vi "CODMn启动命令 (子VI).vi"(9 "强制切换":bool, 10 "CODMn量程切换":enum32{"H", "L", "AUTO"}(ring)=enum."AUTO", 11 "启动测量模式":T1) -> ()   [LabVIEW 2016, in "斯坦道CODMn.lvlib"]
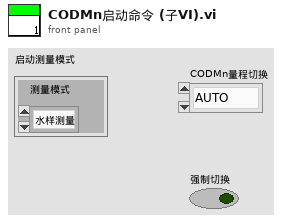
[diagram p1: front panel]
types:
  T1 = cluster{"测量模式":enum16{"水样测量", "标样核查", "零点核查", "跨度核查", "空白测试", "加标回收", "平行样", "校零", "校标"}}
  T2 = cluster{"命令":string, "测量模式":enum16{"水样测量", "标样核查", "零点核查", "跨度核查", "空白测试", "加标回收", "平行样", "校零", "校标"}, "CODMn量程切换":enum32{"H", "L", "AUTO"}}
  T3 = enum16{"水样测量", "标样核查", "零点核查", "跨度核查", "空白测试", "加标回收", "平行样", "校零", "校标"}
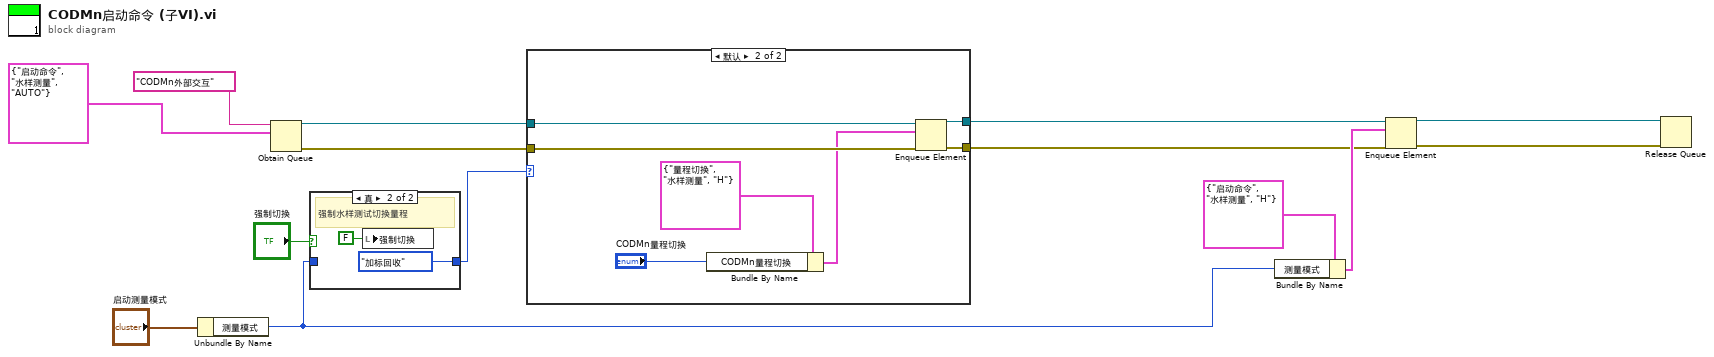
[diagram p0: block diagram]
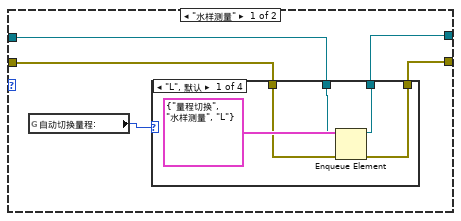
[diagram p3: hidden frame]
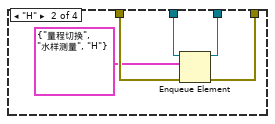
[diagram p4: hidden frame]
diagram:
  n1 = Unbundle By Name("启动测量模式") -> ("测量模式"=w2:T3)
  n2 = Obtain Queue(name (unnamed)="CODMn外部交互" ("名称（未命名）"), element data type=T2 {"命令"="启动命令", "测量模式"=enum."水样测量", "CODMn量程切换"=enum."AUTO"} ("元素")) -> (queue out=w7:refnum<queue>, error out=w6:errorcluster)  [unwired: 3 in, 1 out]
  n3 = case shown="真" "强制切换" {
    tunnel: w2 -> [w15 _]
    tunnel: [w15 T3."加标回收" ("测量模式")] -> w1
    frame False {
    }
    frame True {
      # "强制水样测试切换量程"
      n4 = local write "强制切换"(FALSE ("强制切换")) -> ()
    }
  }
  n5 = case shown="默认" w1 {
    tunnel: w7 -> [w21 w43]
    tunnel: w6 -> [w19 w42]
    tunnel: [w20 w41] -> w5
    tunnel: [w18 w40] -> w4
    frame "水样测量" {
      n6 = global read "CODMn断电保存全局变量.vi" "自动切换量程:"() -> (w22:enum16{"L", "H", "自动切换测一次", "自动切换测两次"})
      n7 = case shown="\"L\", 默认" w22 {
        tunnel: w21 -> [w26 w32 w33 w36]
        tunnel: [w24 w31 w33 w36] -> w20
        tunnel: w19 -> [w25 w30 w34 w35]
        tunnel: [w23 w29 w34 w35] -> w18
        frame "L", Default {
          n8 = Enqueue Element(queue=w26, element=T2 {"命令"="量程切换", "测量模式"=enum."水样测量", "CODMn量程切换"=enum."L"} ("元素"), error in (no error)=w25) -> (queue out=w24:refnum<queue>, error out=w23:errorcluster)  [unwired: 1 in, 1 out]
        }
        frame "H" {
          n9 = Enqueue Element(queue=w32, element=T2 {"命令"="量程切换", "测量模式"=enum."水样测量", "CODMn量程切换"=enum."H"} ("元素"), error in (no error)=w30) -> (queue out=w31:refnum<queue>, error out=w29:errorcluster)  [unwired: 1 in, 1 out]
        }
        frame "自动切换测一次" {
        }
        frame "自动切换测两次" {
        }
      }
    }
    frame Default {
      n10 = Bundle By Name(cluster=T2 {"命令"="量程切换", "测量模式"=enum."水样测量", "CODMn量程切换"=enum."H"} ("元素"), "CODMn量程切换"="CODMn量程切换") -> (w38:T2)
      n11 = Enqueue Element(queue=w43, element=w38, error in (no error)=w42) -> (queue out=w41:refnum<queue>, error out=w40:errorcluster)  [unwired: 1 in, 1 out]
    }
  }
  n12 = Bundle By Name(cluster=T2 {"命令"="启动命令", "测量模式"=enum."水样测量", "CODMn量程切换"=enum."H"} ("元素"), "测量模式"=w2) -> (w8:T2)
  n13 = Enqueue Element(queue=w5, element=w8, error in (no error)=w4) -> (queue out=w12:refnum<queue>, error out=w11:errorcluster)  [unwired: 1 in, 1 out]
  n14 = Release Queue(queue=w12, error in (no error)=w11) -> ()  [unwired: 1 in, 3 out]
